vi "calculatePsrrExtractTone.vi"(6 "Time signal(s) in":waveform(dbl)[](array[waveform]), 8 "error in (no error)":errorcluster, 9 "Calculation method":enum16{"RMS", "Peak-to-peak"}(ring), 10 "Search frequency":dbl, 11 "Instrument handle":refnum<k15>) -> (0 "error out":errorcluster, 1 "Detected wfm parameters":T2, 2 "PSRR":dbl, 3 "Instrument handle out":refnum<k15>, 4 "Detected signal(s)":T1(array[cluster]) {"exported spectrum (dB)"."dB Spectrum (Hann)" format="%.2p"; "exported spectrum (dB)"."df" format="%.2p"; "exported spectrum (dB)"."f0" format="%.2p"})   [LabVIEW 2020]
uses:
  <vilib>/measure/matone.llb/Extract Single Tone Information N Chan.vi
  <vilib>/measure/madcrms.llb/Basic Averaged DC-RMS for N Chan.vi
  <vilib>/measure/mascope.llb/Amplitude and Levels N chan.vi
  <vilib>/measure/NI_MAPro.lvlib
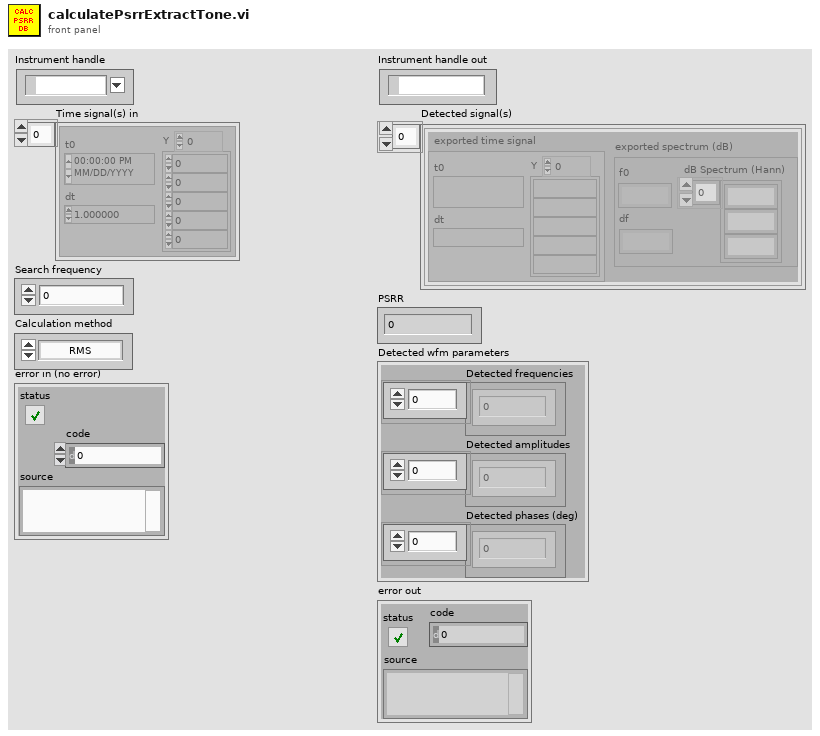
[diagram p1: front panel]
types:
  T1 = cluster{"exported time signal":waveform(dbl), "exported spectrum (dB)":cluster{"f0":dbl, "df":dbl, "dB Spectrum (Hann)":dbl[]}}[]
  T2 = cluster{"Detected frequencies":dbl[], "Detected amplitudes":dbl[], "Detected phases (deg)":dbl[]}
  T3 = enum32{"none", "input signal", "detected signal", "residual signal"}
  T4 = cluster{"Search frequency":dbl, "search (+/- % of Fsampl.)":dbl}
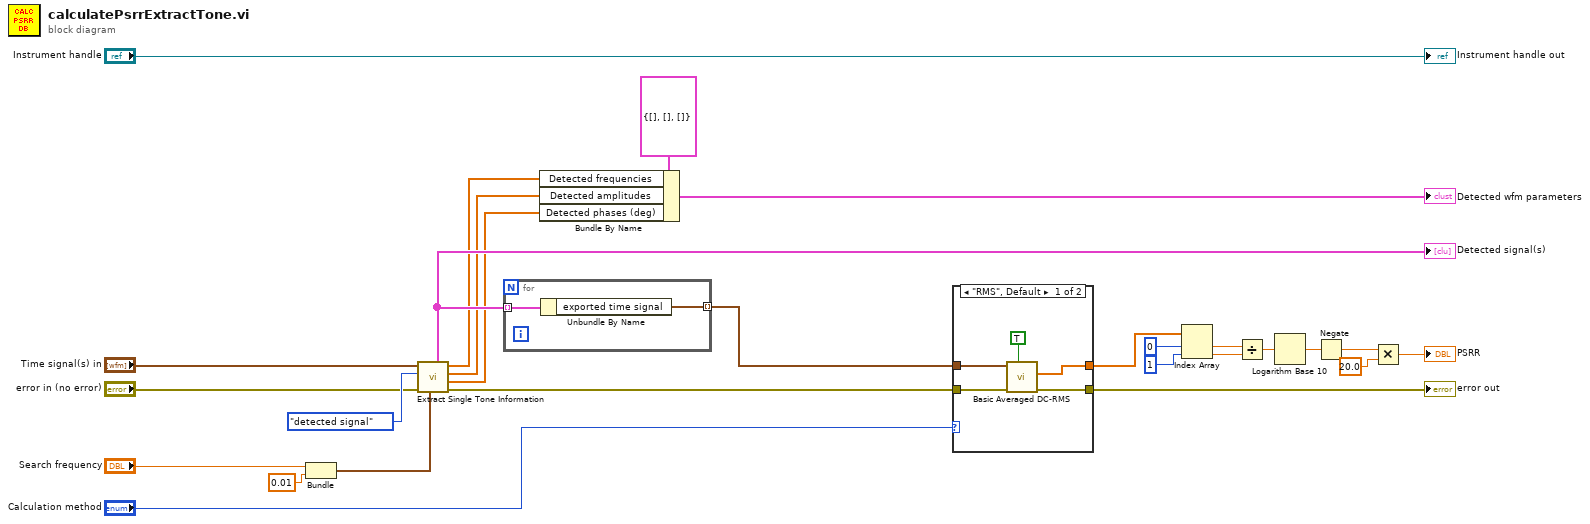
[diagram p0: block diagram]
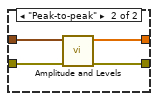
[diagram p2: hidden frame]
diagram:
  n1 = Bundle("Search frequency"="Search frequency", "search (+/- % of Fsampl.)"=0.01) -> (w24:T4)  [unwired: 1 in]
  n2 = call-poly <vilib>:"Extract Single Tone Information.vi"("advanced search"=w24, "error in (no error)"="error in (no error)", "export mode"=T3."detected signal", "time signals in"="Time signal(s) in") -> ("error out"=w15:errorcluster, "detected phases (deg)"=w20:dbl[], "detected amplitudes"=w21:dbl[], "detected frequencies"=w22:dbl[], "exported signals"=w26:T1)  [unwired: 2 in, 1 out]
  "Detected signal(s)" <- w26
  n3 = for {
    tunnel: w26 -> [w29] mode=indexing
    tunnel: [w28] -> w13 mode=indexing
    n4 = Unbundle By Name(w29) -> ("exported time signal"=w28:waveform(dbl))
  }
  n5 = Bundle By Name(cluster=T2 {"Detected frequencies"=[], "Detected amplitudes"=[], "Detected phases (deg)"=[]} ("input cluster"), "Detected frequencies"=w22, "Detected amplitudes"=w21, "Detected phases (deg)"=w20) -> (→"Detected wfm parameters":T2)
  n6 = case shown="\"RMS\", Default" "Calculation method" {
    tunnel: w15 -> [w34 w37]
    tunnel: [w33 w35] -> w14
    tunnel: w13 -> [w32 w38]
    tunnel: [w30 w36] -> w12
    frame "RMS", Default {
      n7 = call-poly <vilib>:"Basic Averaged DC-RMS.vi"("reset"=TRUE, "error in (no error)"=w34, "signals in"=w32) -> ("error out"=w33:errorcluster, "RMS values"=w30:dbl[])  [unwired: 5 in, 2 out]
    }
    frame "Peak-to-peak" {
      n8 = call-poly <vilib>:"Amplitude and Levels.vi"("error in (no error)"=w37, "signal(s) in"=w38) -> ("error out"=w35:errorcluster, "amplitude"=w36:dbl[])  [unwired: 6 in, 2 out]
    }
  }
  "error out" <- w14
  n9 = Index Array(array=w12, index #1=0 ("index"), index #2=1 ("index")) -> (element #1=w8:dbl, element #2=w9:dbl)
  n10 = Divide(x=w8, y=w9) -> (x/y=w7:dbl)
  n11 = Logarithm Base 10(1:w7) -> (0:w6:dbl)
  n12 = Negate(x=w6) -> (-x=w2:dbl)
  n13 = Multiply(x=w2, y=20.0) -> (x*y=→"PSRR":dbl)
  "Instrument handle out" <- "Instrument handle"
